vi "SteuerungWaermepumpe - Kopie_11.01.17.vi"() -> ()   [LabVIEW 2015]
uses:
  <vilib>/DAQmx/read.llb/DAQmx Read (Analog 1D Wfm NChan NSamp).vi
  <vilib>/DAQmx/write.llb/DAQmx Write (Analog 1D Wfm NChan 1Samp).vi
  <vilib>/MakerHub/LINX/Public/Peripherals/Digital/Digital Write N Chans.vi
  <vilib>/MakerHub/LINX/Private/Local IO/LinxDigitalWrite.vi
  <vilib>/MakerHub/LINX/Public/Utilities/Check Channel.vi
  <vilib>/MakerHub/LINX/Private/Utilties/Generate Error.vi
  <vilib>/DAQmx/miscellaneous.llb/DAQmx Fill In Error Info.vi
  <vilib>/Utility/file.llb/Read Delimited Spreadsheet (DBL).vi
  <vilib>/MakerHub/LINX/LMH-LINX.lvlib
panel:
  out "Array 2":waveform(dbl)[](array[waveform])
  in  "Messplatten speichern":bool caption="Enable"
  in  "Wartezeit 2":u32=500
  in  "Wartezeit 1":u32=9000
  out "Abscheider":cluster{dbl, dbl, dbl}(slide) scale=0.0..1.3
  in  "Rampe":bool=TRUE
  in  "Rampe rpm/s":dbl=1.0 min=1.0 max=100.0 step=1.0
  out "Rampe IW":dbl
  in  "reinitialize HD":bool
  in  "reinitialize Pumpe":bool
  out "ist an!":string
  in  "zusätzlicher Druck":dbl
  in  "PI05 SW":dbl format="%.2f"
  out "p_liq_mittel":dbl
  out "p_liq":dbl
  out "Schleifendauer":dbl format="%.5f"
  out "Mittelwert 2":dbl
  in  "Mittelwert HD":bool
  in  "Mittelwert Pumpe":bool
  out "Mittelwert":dbl
  in  "Xi / p_liq berechnung an":bool
  out "xi_r":dbl
  in  "Regler Senke":bool
  in  "reinitialize Senke":bool
  in  "TI35 SW":dbl=43.0 format="%.2f"
  in  "Drehzahl Bestätigung":bool
  in  "Drehzahl SW":dbl=1000.0 min=500.0 max=3000.0 step=1.0 format="%#_4g"
  out "Check":dbl format="%#_13g"
  in  "Regler Hochdruck":bool
  in  "PID Regelung Pumpe":bool
  in  "SW TI39":dbl
  out "Array":bool[](array[boolean])
  in  "LEDs 2":bool[](array[boolean])
  in  "Regelung HK":bool
  in  "RV 30 zu":bool
  in  "RV 30 auf":bool
  out "FI_Oel":dbl
  in  "RV 33":dbl(slide) scale=-1.0..1.0
  in  "tag":string
  out "Pumpenwerte":dbl[](array[numeric]) format="%.2f"
  out "Speichert!":bool
  out "Historie":string
  in  "Kommentar":string
  out "refnum out":refnum<file>
  in  "Identität!":string(combo)
  in  "Zeit X in Minuten":dbl(slide)=5.0 min=0.0 max=15.0 scale=5.0..15.0
  out "TI 21a Warnungen":dbl
  out "Leistung":dynamicdata(graph)
  out "TI 37":dbl
  in  "Programm stoppen!":bool
  out "%":sgl(slide) scale=0.0..100.0
  out "kalt":bool
  out "warm":bool
  out "?":T1(array[cluster]) {"?" format="%#.4g"; "Konzentration_reich" format="%#.4g"}
  in  "Mit EES vergleichen":bool
  in  "FI13 SW in l/min":dbl=3.0 min=3.0 max=12.0 step=0.10000000149011612
  out "COP_Oel":dbl
  out "Q-Oel kW":dbl format="%_4g"
  in  "Dateiname!":string
  in  "Comment":bool
  in  "Speichern":bool caption="Aktivieren"
  out "ZU     Ventilstellung 33     AUF":dbl(slide) scale=0.0..100.0 scale format="%.2f"
  in  "Regelventil 34":dbl(slide) min=0.0 max=100.0 step=0.009999999776482582 scale=0.0..100.0
  in  "Matlab":bool
  in  "?":T2(tab)
  out "?":dynamicdata(graph)
  out "?":waveform(dbl)(graph)
  out "?":dynamicdata(graph)
  out "PI 12":dbl format="%.2f"
  out "PI 11":dbl format="%.2f"
  out "Dichte":dbl format="%.5g"
  in  "Reset":bool
  out "Betriebszeit":cluster{"second":i32, "minute":i32, "hour":i32}
  out "Temperatur Ölprüfstand":dbl
  out "FI 13 kg/min":dbl
  in  "Messung\nFrequenzwandler":bool
  out "Magnetventil":bool
  out "Fl.Pumpe an":bool
  out "Temperatur Öl":bool
  out "COP":dbl format="%#_13g"
  out "Verdichteraktivität":cluster{"second":i32, "minute":i32, "hour":i32}
  out "Q-Entgaser kW":dbl format="%_4g"
  out "Warnungen":bool[](array[boolean])
  out "Status Komponenten":bool[](array[boolean])
  in  "Pumpen-Auto-Abschalt":bool=TRUE
  out "Q-Resorber kW":dbl format="%_4g"
  out "Stellung Expansionsventil":waveform(dbl)(graph)
  out "FI 35 l/min":dbl format="%#_13g"
  out "FI 38 l/min":dbl format="%#_13g"
  out "FI Oel l/min":dbl format="%#.3g"
  out "LI in l":dbl format="%#_4g"
  out "TI 39":dbl format="%#_3g"
  out "TI 38":dbl format="%#_3g"
  out "TI 36":dbl format="%#_3g"
  out "TI 35":dbl format="%#_3g"
  out "TI 33":dbl format="%#_3g"
  out "TI 32":dbl format="%#_3g"
  out "TI 34":dbl format="%#_3g"
  out "TI 21a":dbl format="%#_3g"
  out "TI 21":dbl format="%#_3g"
  out "TI 20":dbl format="%#_3g"
  out "TI 14a":dbl format="%#_3g"
  out "TI 14":dbl format="%#_3g"
  out "TI 13":dbl format="%#_3g"
  out "TI 12":dbl format="%#_3g"
  out "TI 11":dbl format="%#_3g"
  out "TI 10":dbl format="%#_3g"
  out "TI 09":dbl format="%#_3g"
  out "TI 08":dbl format="%#_3g"
  out "TI 07":dbl format="%#_3g"
  out "TI 06a":dbl format="%#_3g"
  out "TI 06":dbl format="%#_3g"
  out "TI 05":dbl format="%#_3g"
  out "TI 04":dbl format="%#_3g"
  out "TI 22":dbl format="%#_3g"
  out "TI 02":dbl format="%#_3g"
  out "TI 01":dbl format="%#_3g"
  out "Konzentration":dbl format="%#_5g"
  in  "Pumpensteuerung":dbl min=0.0 max=10.0 step=0.009999999776482582 format="%.2g"
  out "PI 08":dbl format="%.2f"
  out "PI 05":dbl format="%#.2f"
  out "PI 02":dbl format="%.2f"
  out "PI 04":dbl format="%.2f"
  out "PDI 8-9":dbl format="%.2f"
  out "PI 14":dbl format="%.2f"
  out "PI 01":dbl format="%.2f"
  out "ZU    Ventilstellung Exp.V     AUF":dbl(slide) scale=0.0..100.0 scale format="%#.1f"
  in  "Exp.V":dbl(slide)=3.0 min=0.0 max=100.0 step=1.0 scale=0.0..100.0 scale format="%#.0f"
  out "ZU    Ventilstellung 14      AUF":dbl(slide) caption="Auf    Ventilstellung 14      Zu" scale=0.0..100.0 scale format="%#.2f"
  in  "Regelventil 36":dbl(slide) min=0.0 max=100.0 step=0.009999999776482582 scale=0.0..100.0 scale format="%#.0f"
  out "ZU  Ventilstellung 35  AUF":dbl(slide) scale=0.0..100.0 scale format="%.2f"
  in  "Regelventil 35":dbl(slide)=100.0 min=0.0 max=100.0 step=0.009999999776482582 scale=0.0..100.0 scale format="%#.3g"
  out "ZU     Ventilstellung 39     AUF":dbl(slide) scale=0.0..100.0 scale format="%.2f"
  in  "Regelventil 39":dbl(slide)=100.0 min=0.0 max=100.0 step=0.009999999776482582 scale=0.0..100.0
  out "FI 13 l/min":dbl format="%.2f"
  out "FI 07 l/min":dbl format="%.2f"
  out "LI in m":dbl format="%.2f"
  out "PDI 5-6":dbl format="%.4f"
  out "PI 07":dbl format="%.2f"
  out "Druckverhältnis":dbl
  out "Drehzahl":dbl
  out "Drehmoment":dbl
  out "Frequenz":dbl
  out "Leistung":dbl
  out "Durchfluss":waveform(dbl)[](graph)
  in  "Tab Control Temperaturen":T3(tab)
  out "Temperatur Reich":waveform(dbl)[](graph)
  out "Temperatur Arm":waveform(dbl)[](graph)
  out "Temperatur Öl":waveform(dbl)[](graph)
  out "Temperatur Senke/Quelle":waveform(dbl)[](graph)
  out "Druck":waveform(dbl)[](graph)
  out "Druckzustand":bool caption="Zu viel Druck !!!"
  # "Öltemperatur"
  # "Resorber"
  # "Entgaser"
  # "Druckverhältnis"
  # "ExpV"
  # "Verdichter an"
  # "iWÜ"
  # "Magnetventil"
  # "RV 39"
  # "Leer"
  # "RV 33"
  # "RV 35"
  # "RV 34"
  # "Pumpe an"
  # "Ölabscheider"
  # "2"
  # "1"
  # "RV 30"
  # "Verdichter"
  # "Pumpe"
  # "Leistung"
  # "kW"
  # "Speed"
  # "rpm"
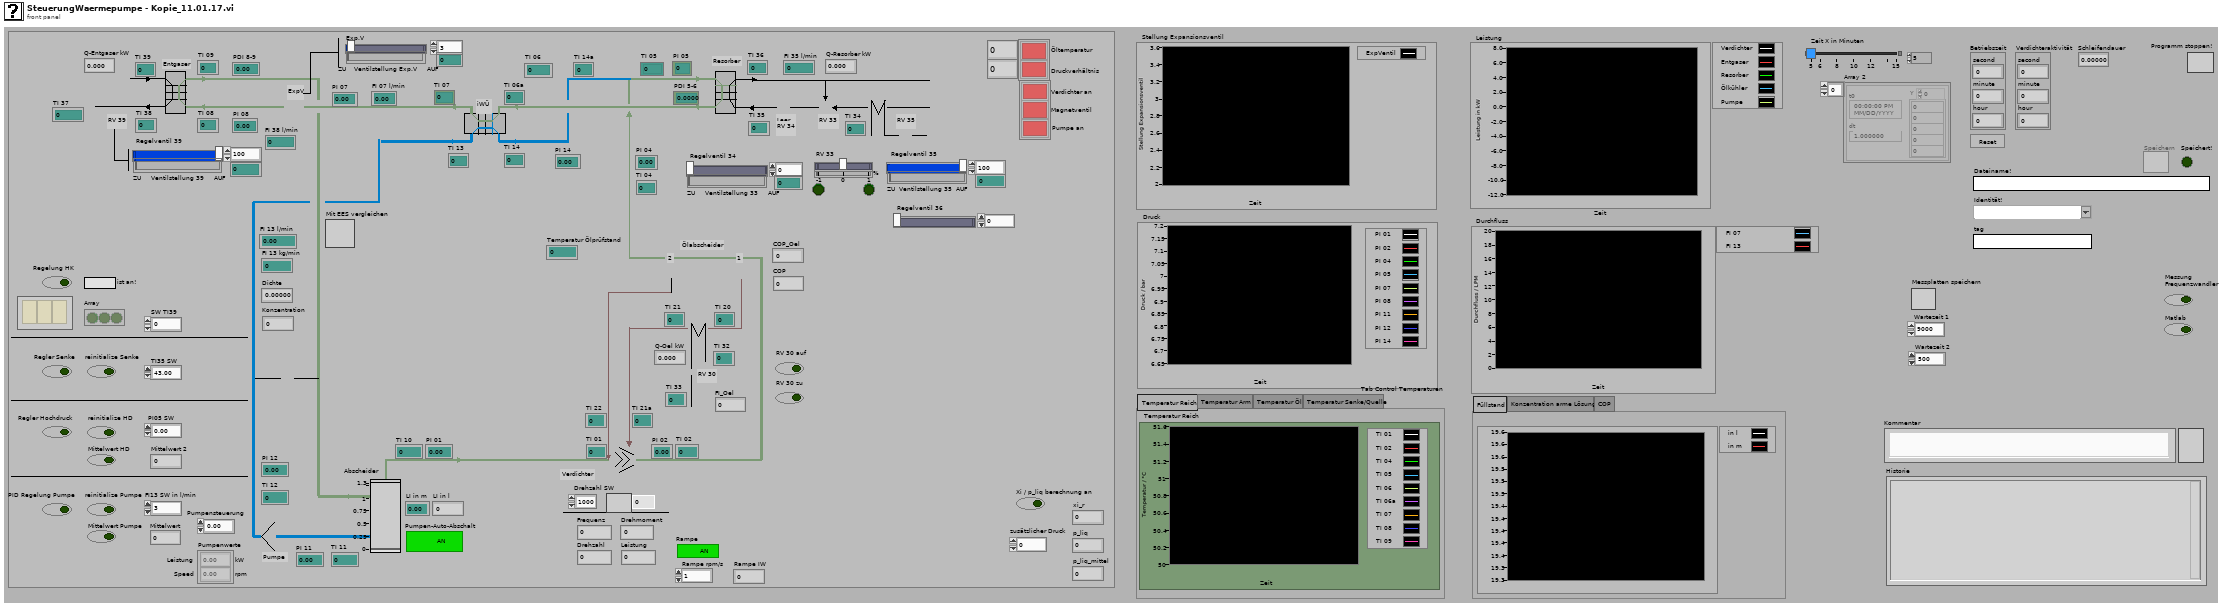
[diagram p1: front panel]
types:
  T1 = cluster{dbl, "Konzentration_reich":dbl, "String":string, bool}[]
  T2 = enum32{"Füllstand", "Konzentration arme Lösung", "COP"}
  T3 = enum32{"Temperatur Reich", "Temperatur Arm", "Temperatur Öl", "Temperatur Senke/Quelle"}
  T4 = enum8{"Enabled", "Disabled", "Disabled and Grayed Out"}
  T5 = typedef "LMH-LINX.lvlib/LINX Ref.ctl" = cluster{"IO":T6, "Interface":T7, "LINX Device Config":T8}
  T6 = typedef "LMH-LINX.lvlib/Platform.ctl" = enum16{"Remote", "Local"}
  T7 = typedef "LMH-LINX.lvlib/Interface.ctl" = enum16{"Serial", "TCP"}
  T8 = typedef "LMH-LINX.lvlib/Device.lvlib/LINX Device Config.ctl" = cluster{"Interface":T7, "COM Port":refnum<visa-resource-name>, "TCP Configuration":T9, "Device Family":u8, "Device ID":u8, "Device Name":string, "TCP Ref":refnum<k5>, "Channels":T10}
  T9 = typedef "LMH-LINX.lvlib/Device.lvlib/TCP Config.ctl" = cluster{"IP Address":string, "Port":u16}
  T10 = typedef "LMH-LINX.lvlib/Channels.ctl" = cluster{"DI":u8[], "DO":u8[], "AI":u8[], "AO":u8[], "PWM":u8[], "QE":u8[], "UART":u8[], "I2C 2":u8[], "SPI":u8[], "CAN":u8[], "Servo":u8[], "AI Ref (V)":dbl, "AI Resolution (Bits)":u8, "AO Ref (V)":dbl, "AO Resolution (Bits)":u8}
  T11 = enum16{"open", "replace", "create", "open or create", "replace or create", "replace or create with confirmation"}
  T12 = cluster{"Array[0]":dbl, "Array[1]":dbl, "Array[2]":dbl}
  T13 = cluster{"Array[0]":sgl, "Array[1]":sgl, "Array[2]":sgl}
  T14 = cluster{"Numeric":dbl, "Konzentration_reich":dbl, "String":string, bool}[]
  T15 = typedef "LVDateTimeRec.ctl" = cluster{"fractional second":dbl, "second":i32, "minute":i32, "hour":i32, "day of month":i32, "month":i32, "year":i32, "day of week":i32, "day of year":i32, "DST":i32}
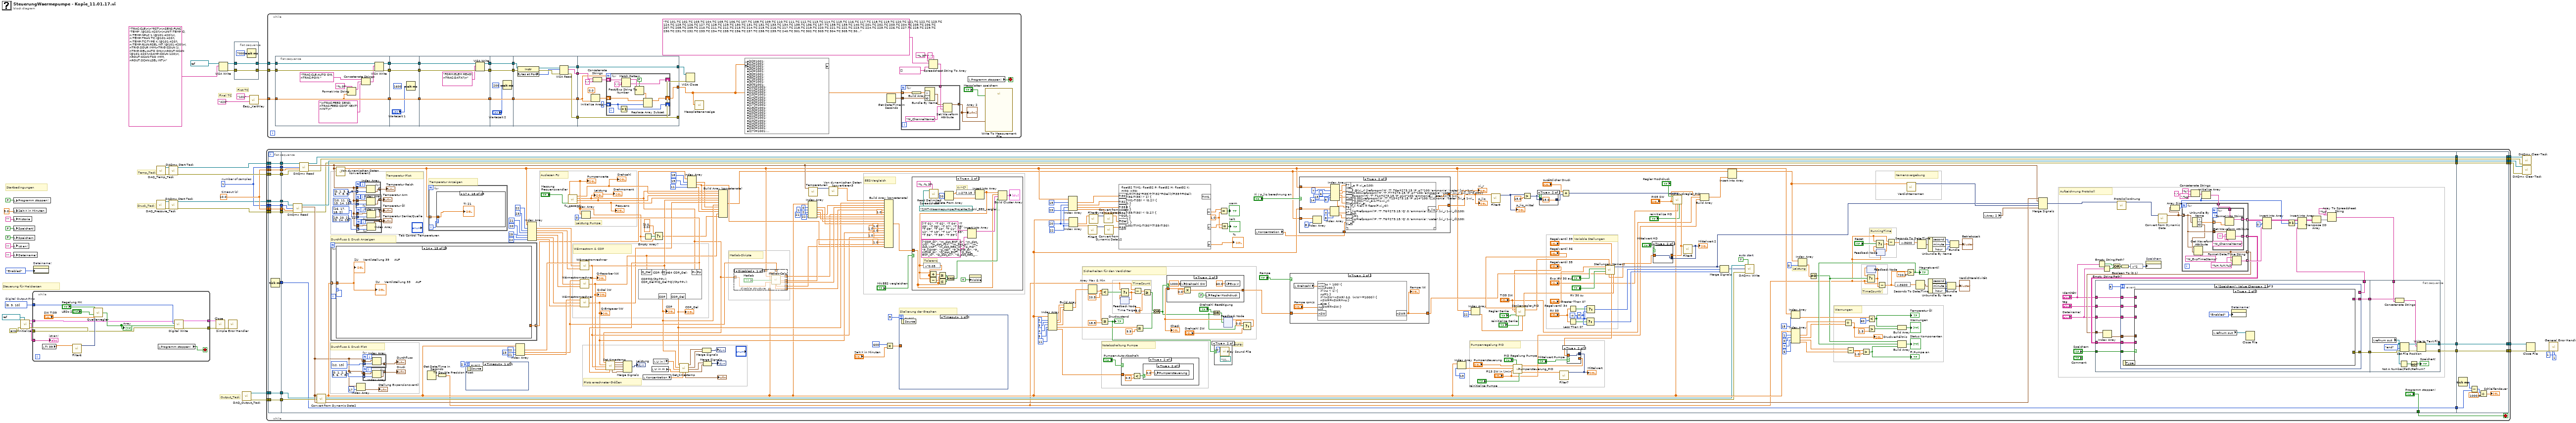
[diagram p0: block diagram]
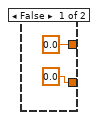
[diagram p8: hidden frame]
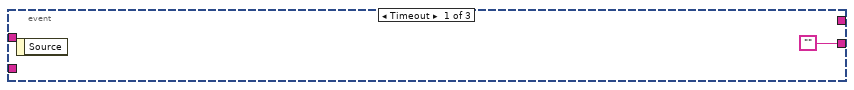
[diagram p10: hidden frame]
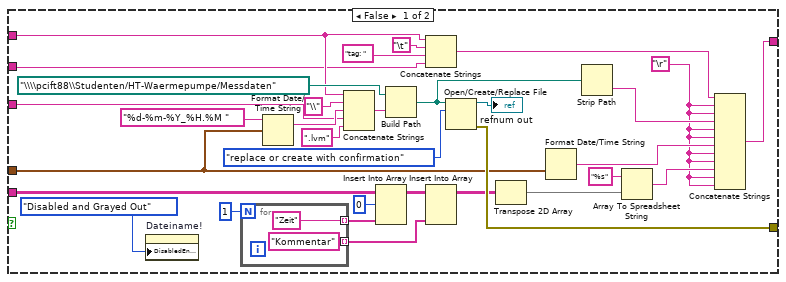
[diagram p11: hidden frame]
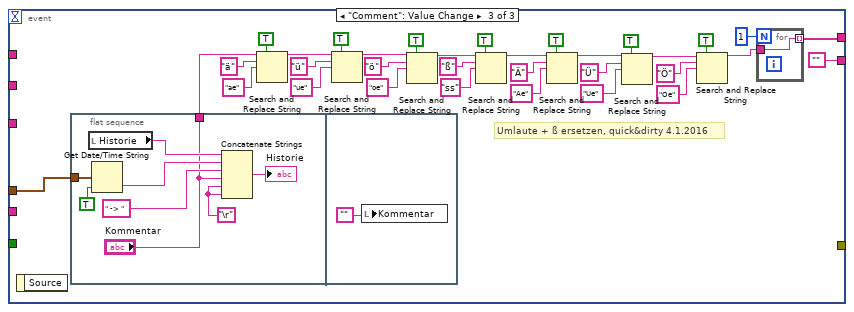
[diagram p12: hidden frame]
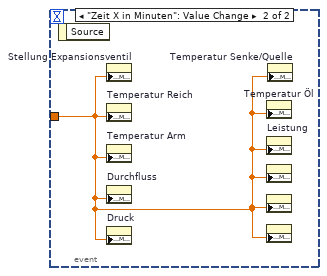
[diagram p13: hidden frame]
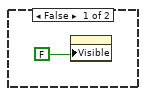
[diagram p14: hidden frame]
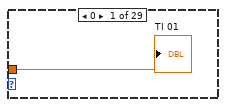
[diagram p17: hidden frame]
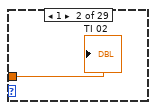
[diagram p18: hidden frame]
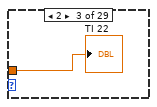
[diagram p19: hidden frame]
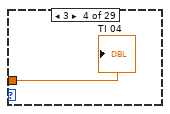
[diagram p20: hidden frame]
diagram:
  w19 = 10.0  # timeout (s)
  w18 = 1  # number of samples
  w31 = i32[] [8, 9, 10]  # Digital Output PIns
  # "Final TC"
  # "First TC"
  # "Output_Task"
  # "Druck_Task"
  # "Temp_Task"
  # "Steuerung für Heizkerzen"
  # "Startbedingungen"
  n1 = local write "Programm stoppen!"(FALSE ("Programm stoppen!")) -> ()
  n2 = local write "Zeit X in Minuten"(5.0 ("Zeit X in Minuten")) -> ()
  n3 = local write "Historie"("") -> ()
  n4 = local write "Speichert!"(FALSE ("Speichert!")) -> ()
  n5 = local write "Speichern"(FALSE ("Speichern")) -> ()
  n6 = local write "ist an!"("") -> ()
  n7 = local write "Dateiname!"("") -> ()
  n8 = call <vilib>:"Initialize.vi"("Serial Port"=refnum<visa-resource-name> "COM4", "Error In"=errorcluster {"status"=FALSE, "code"=0, "source"=""}) -> ("Error Out"=w32:errorcluster, "Device Name"=w29:string, "LINX Resource"=w35:T5)  [unwired: 7 in]
  n9 = while {
    tunnel: w35 -> [w50]
    tunnel: [w60] -> w34
    tunnel: [w59] -> w33
    tunnel: w32 -> [w49]
    tunnel: w31 -> [w58]
    tunnel: w29 -> [w48]
    stop <- w57 stop-if-true
    n10 = local read "TI 39"() -> (w51:dbl)
    n11 = call "Filter6"("Signal"=w51) -> ("Filtered Signal"=w52:dynamicdata)  [unwired: 9 in, 1 out]
    n12 = call "Quellenregler.vi"("Regelung Quelle"="Regelung HK", "TI 38 IW °C"=w52, "LEDs"="LEDs 2", "TI 38 SW °C"="SW TI39") -> ("Kerzen von Regler"=w54:bool[])  [unwired: 3 in, 1 out]
    "Array" <- w54
    n13 = local read "Programm stoppen!"() -> (w57:bool)
    n14 = call-poly <vilib>:"Digital Write.vi"("Error In"=w49, "Values"=w54, "DO Channels"=w58, "LINX Resource"=w50) -> ("Error Out"=w59:errorcluster, "LINX Resource"=w60:T5)  [unwired: 6 in]
    "ist an!" <- w48
  }
  n15 = property on="Dateiname!" class="Str"("DisabledEnum"=T4."Enabled" ("Disabled")) -> ()  [unwired: 2 in, 2 out]
  n16 = call "DAQ_Pressure_Task.vi"() -> ("error out"=w23:errorcluster, "task out"=w24:refnum<k21>)  [unwired: 10 in]
  n17 = call "DAQ_Temp_Task.vi"() -> ("error out"=w25:errorcluster, "task out"=w26:refnum<k21>)  [unwired: 10 in]
  n18 = call <vilib>:"DAQmx Start Task.vi"("task/channels in"=w24, "error in"=w23) -> ("task out"=w17:refnum<k21>, "error out"=w20:errorcluster)  [unwired: 12 in]
  n19 = call <vilib>:"DAQmx Start Task.vi"("task/channels in"=w26, "error in"=w25) -> ("task out"=w21:refnum<k21>, "error out"=w22:errorcluster)  [unwired: 12 in]
  n20 = call <vilib>:"Close.vi"("Error In"=w33, "LINX Resource"=w34) -> ("Error Out"=w36:errorcluster)  [unwired: 9 in]
  n21 = VISA Write(VISA resource name=refnum<visa-resource-name> "COM3", write buffer="TRAC:CLE\n\n*RST\n\nSENS:FUNC 'TEMP',(@101:420)\n\nUNIT:TEMP C\n:TEMP:NPLC 1,(@101:420)\n\n:TEMP:TRAN TC,(@101:420)\n:TEMP:TC:TYPE K,(@101:420)\n:TEMP:RJUN:RSEL INT,(@101:420)\n\nTRIG:SOUR IMM\nTRIG:COUN 1\nTRIG:DEL:AUTO ON\n\nROUT:SCAN  (@101:420)\nSAMP:COUN 120\n\nROUT:SCAN:TSO IMM\nROUT:SCAN:LSEL INT\n") -> (VISA resource name out=w5:refnum<visa-resource-name>, error out=w6:errorcluster)  [unwired: 1 in, 1 out]
  n22 = call <vilib>:"Simple Error Handler.vi"("error in (no error)"=w36) -> ()  [unwired: 4 in, 5 out]
  n23 = flat-sequence {
    tunnel: w6 -> [w63]
    tunnel: [w63] -> w3
    tunnel: w5 -> [w61]
    tunnel: [w61] -> w4
    frame #0 {
      n24 = Wait (ms)(milliseconds to wait=u32 7000 ("Zu wartende ms")) -> ()  [unwired: 1 out]
    }
  }
  n25 = call "DAQ_Output_Task.vi"() -> ("error out"=w11:errorcluster, "task out"=w12:refnum<k21>)  [unwired: 10 in]
  n26 = call "Easy_Keithley.vi"("Final Thermocouple ID# (String)"="420", "First Thermocouple ID# (String)"="101") -> ("Number of Thermocouples"=w7:dbl)  [unwired: 8 in, 1 out]
  n27 = while {
    tunnel: [w98] -> w41
    tunnel: [w97] -> w40
    tunnel: w22 -> [w91]
    tunnel: w19 -> [w89]
    tunnel: w21 -> [w86]
    tunnel: w18 -> [w84]
    tunnel: w20 -> [w82]
    tunnel: w19 -> [w81]
    tunnel: w18 -> [w79]
    tunnel: w17 -> [w77]
    tunnel: [w73] -> w16
    tunnel: [w72] -> w15
    tunnel: [w70] -> w14
    tunnel: [w68] -> w13
    tunnel: w12 -> [w67]
    tunnel: w11 -> [w64]
    stop <- w96 stop-if-true
    n28 = flat-sequence {
      tunnel: [w109] -> w92
      tunnel: w91 -> [w108]
      tunnel: [w108] -> w90
      tunnel: w89 -> [w107]
      tunnel: [w107] -> w88
      tunnel: w86 -> [w106]
      tunnel: [w106] -> w87
      tunnel: [w105] -> w85
      tunnel: w84 -> [w105]
      tunnel: [w104] -> w83
      tunnel: w82 -> [w104]
      tunnel: w81 -> [w103]
      tunnel: [w103] -> w80
      tunnel: w79 -> [w102]
      tunnel: [w102] -> w78
      tunnel: w77 -> [w101]
      tunnel: [w101] -> w76
      tunnel: w67 -> [w100]
      tunnel: [w100] -> w66
      tunnel: [w99] -> w65
      tunnel: w64 -> [w99]
      tunnel: ["Programm stoppen!"] -> w96
      tunnel: [w327] -> w95
      tunnel: [w326] -> w94
      tunnel: [w131] -> w93
      tunnel: w92 -> [w131]
      tunnel: w90 -> [w168]
      tunnel: w88 -> [w167]
      tunnel: w87 -> [w166]
      tunnel: w85 -> [w165]
      tunnel: w83 -> [w164]
      tunnel: w80 -> [w163]
      tunnel: w78 -> [w162]
      tunnel: w76 -> [w161]
      tunnel: [w160] -> w75
      tunnel: [w159] -> w74
      tunnel: [w158] -> w71
      tunnel: [w157] -> w69
      tunnel: w66 -> [w155]
      tunnel: w65 -> [w154]
      tunnel: [w738] -> w97
      tunnel: [w739] -> w98
      tunnel: w95 -> [w739]
      tunnel: w94 -> [w738]
      tunnel: w93 -> [w736]
      tunnel: w75 -> [w731]
      tunnel: w74 -> [w732]
      tunnel: [w732] -> w73
      tunnel: [w731] -> w72
      tunnel: w71 -> [w730]
      tunnel: [w730] -> w70
      tunnel: w69 -> [w729]
      tunnel: [w729] -> w68
      frame #0 {
        n29 = Tick Count (ms)() -> (millisecond timer value=w109:u32)
      }
      frame #1 {
        w133 = 8.0  # Time Target
        w156 = TRUE  # auto start
        w347 = sgl 1.0
        w360 = 22
        w365 = 20
        w391 = -4
        w392 = 0
        # "RunningTime"
        # "TimeCountV"
        # "TimeCount"
        # "ENTE!"
        # "Sicherheiten für den Verdichter"
        # "Pumpenregelung PID"
        # "Skalierung der Graphen"
        # "Leistung Pumpe"
        # "Leistung"
        # "Durchfluss & Druck Anzeigen"
        # "Temperatur Anzeigen"
        # "Plots errechneter Größen"
        # "EES-Vergleich"
        # "Matlab-Skripte"
        # "Warnungen"
        # "Namensvergebung"
        # "Wärmestrom & COP"
        # "Notabschaltung Pumpe"
        # "Auslesen FU"
        # "Durchfluss & Druck Plot"
        # "Temperatur Plot"
        # "Aufzeichnung Protokoll"
        # "Variable Stellungen"
        n30 = call-poly <vilib>:"DAQmx Read.vi"("task/channels in"=w161, "number of samples per channel"=w162, "timeout"=w163, "error in"=w164) -> ("task out"=w160:refnum<k21>, "data"=w170:waveform(dbl)[], "error out"=w157:errorcluster)  [unwired: 9 in]
        n31 = call-poly <vilib>:"DAQmx Read.vi"("task/channels in"=w166, "number of samples per channel"=w165, "timeout"=w167, "error in"=w168) -> ("task out"=w159:refnum<k21>, "data"=w169:waveform(dbl)[], "error out"=w158:errorcluster)  [unwired: 9 in]
        n32 = call "Convert from Dynamic Data2"("Dynamic Data Type"=w170) -> ("Array"=w175:dbl[])  [unwired: 3 in]
        n33 = for {
          tunnel: w175 -> [w677] mode=indexing
          tunnel: [w676] -> w180 mode=indexing
          i -> [w678]
          n34 = case shown="14" w678 {
            tunnel: w677 -> [w679 w680 w681 w682 w683 w684 w685 w686 w687 w688 w689 w698 w710 w713 w714 w715 w716 w717 w720 w724 w725 w726 w727 w728 _]
            tunnel: [_ _ _ _ _ _ _ _ _ _ _ w690 _ _ _ _ _ _ w718 w722 _ _ _ _ _] -> w676
            frame 0 {
              "PI 01" <- w679
            }
            frame 1 {
              "PI 02" <- w680
            }
            frame 2 {
              "PI 04" <- w681
            }
            frame 3 {
              "PI 05" <- w682
            }
            frame 4 {
              "PI 07" <- w683
            }
            frame 5 {
              "PI 08" <- w684
            }
            frame 6 {
              "PI 11" <- w685
            }
            frame 7 {
              "PI 12" <- w686
            }
            frame 8 {
              "PI 14" <- w687
            }
            frame 9 {
              "PDI 5-6" <- w688
            }
            frame 10 {
              "PDI 8-9" <- w689
            }
            frame 11 {
              n35 = call "Filter3"("Signal"=w698) -> ("Filtered Signal"=w696:dynamicdata)  [unwired: 9 in, 1 out]
              n36 = Greater?(x=w698, y=0.3) -> (0:w693:bool)
              n37 = case shown="False" w693 {
                tunnel: w698 -> [_ w709]
                tunnel: [0.0 w709] -> w701
                frame False {
                }
                frame True {
                }
              }
              n38 = call "Convert from Dynamic Data6"("Dynamic Data Type"=w696) -> ("Scalar"=w695:dbl)  [unwired: 3 in]
              n39 = Multiply(x=w695, y=10.0) -> (x*y=w697:dbl)
              n40 = Greater?(x=w698, y=0.4) -> (0:w694:bool)
              n41 = formula code="float64 y; float64 Vu; /*Vu: Volumen schmaler Zylinder+Fuellstandsmesser*/\nVu=10;  /* 10 Liter */\n\nif (x<=10.25) \ny=(x-1)*pi*(0.536**2+0.32**2);\nelse\ny=Vu+(x-10.25)*pi*(1.584**2+0.32**2);"("x"=w697) -> ("y"=w690:dbl)
              "LI in l" <- w690
              n42 = case shown="False" w694 {
                tunnel: w698 -> [_ w707]
                tunnel: [0.0 w707] -> w700
                frame False {
                }
                frame True {
                }
              }
              n43 = Merge Signals(w698, w701, w700) -> (w702:dynamicdata)
              n44 = call "Convert from Dynamic Data3"("Dynamic Data Type"=w702) -> ("Array"=w705:dbl[])  [unwired: 3 in]
              n45 = Array To Cluster(array=w705) -> (cluster=w692:T12)
              n46 = To Single Precision Float(number=w692) -> (single precision float=→"Abscheider":T13)
              "LI in m" <- w698
            }
            frame 12 {
              "FI 07 l/min" <- w710
            }
            frame 13 {
              n47 = local read "Dichte"() -> (w712:dbl)
              n48 = Multiply(x=w713, y=w712) -> (x*y=→"FI 13 kg/min":dbl)
              "FI 13 l/min" <- w713
            }
            frame 14 {
              "ZU     Ventilstellung 39     AUF" <- w714
              "ZU     Ventilstellung 33     AUF" <- w714
            }
            frame 15 {
              "ZU  Ventilstellung 35  AUF" <- w715
            }
            frame 16 {
              # "RV14 ist entfernt"
              "ZU    Ventilstellung 14      AUF" <- w716
            }
            frame 17 {
              "ZU    Ventilstellung Exp.V     AUF" <- w717
            }
            frame 18 {
              n49 = call "Filter"("Signal"=w720) -> ("Filtered Signal"=w719:dynamicdata)  [unwired: 9 in, 1 out]
              n50 = call "Convert from Dynamic Data4"("Dynamic Data Type"=w719) -> ("Scalar"=w721:dbl)  [unwired: 3 in]
              n51 = formula code="float64 D;\nD=9.375*StromDichte+0.7125;\nD=floor(D*100000)/100000;"("StromDichte"=w721) -> ("D"=w718:dbl)
              "Dichte" <- w718
            }
            frame 19 {
              n52 = call "Filter2"("Signal"=w724) -> ("Filtered Signal"=w723:dynamicdata)  [unwired: 9 in, 1 out]
              n53 = To Double Precision Float(number=w723) -> (double precision float=w722:dbl)
              "Konzentration" <- w722
            }
            frame 20 {
              "FI Oel l/min" <- w725
            }
            frame 21 {
              "FI 38 l/min" <- w726
            }
            frame 22 {
              "FI 35 l/min" <- w727
            }
            frame 23 {
              "FI_Oel" <- w728
            }
            frame 24, Default {
            }
          }
        }
        n54 = call "Von dynamischen Daten konvertieren2"("Dynamic Data Type"=w169) -> ("Array"=w116:dbl[])  [unwired: 3 in]
        n55 = for {
          tunnel: i32[] [0, 1, 3, 4, 5, 6, 7, 8, 9] -> [w491] mode=indexing
          tunnel: w169 -> [w490]
          tunnel: [w489] -> w263 mode=indexing
          n56 = Index Array(array=w490, index=w491) -> (element=w489:waveform(dbl))
        }
        "Temperatur Reich" <- w263
        n57 = for {
          tunnel: i32[] [10, 11, 12, 13, 14, 15] -> [w488] mode=indexing
          tunnel: w169 -> [w487]
          tunnel: [w486] -> w264 mode=indexing
          n58 = Index Array(array=w487, index=w488) -> (element=w486:waveform(dbl))
        }
        "Temperatur Arm" <- w264
        n59 = for {
          tunnel: i32[] [16, 17, 18, 2] -> [w485] mode=indexing
          tunnel: w169 -> [w484]
          tunnel: [w483] -> w265 mode=indexing
          n60 = Index Array(array=w484, index=w485) -> (element=w483:waveform(dbl))
        }
        "Temperatur Öl" <- w265
        n61 = Index Array(array=w170, index=17) -> (element=→"Stellung Expansionsventil":waveform(dbl))
        n62 = for {
          tunnel: i32[] [19, 20, 21, 22, 23, 24, 25] -> [w482] mode=indexing
          tunnel: w169 -> [w481]
          tunnel: [w480] -> w266 mode=indexing
          n63 = Index Array(array=w481, index=w482) -> (element=w480:waveform(dbl))
        }
        "Temperatur Senke/Quelle" <- w266
        n64 = for {
          tunnel: [w476] -> w261 mode=indexing
          tunnel: w170 -> [w475]
          tunnel: i32[] [0, 1, 2, 3, 4, 5, 6, 7, 8] -> [w474] mode=indexing
          n65 = Index Array(array=w475, index=w474) -> (element=w476:waveform(dbl))
        }
        "Druck" <- w261
        n66 = for {
          tunnel: [w479] -> w262 mode=indexing
          tunnel: w170 -> [w478]
          tunnel: i32[] [12, 13] -> [w477] mode=indexing
          n67 = Index Array(array=w478, index=w477) -> (element=w479:waveform(dbl))
        }
        "Durchfluss" <- w262
        n68 = Get Date/Time In Seconds() -> (seconds since 1Jan1904=w130:timestamp)
        n69 = for {
          tunnel: w116 -> [w646] mode=indexing
          i -> [w647]
          n70 = case shown="17" w647 {
            tunnel: w646 -> [w648 w649 w650 w651 w652 w653 w654 w655 w656 w657 w658 w659 w660 w661 w662 w663 w664 w665 w666 w667 w668 w669 w670 w671 w672 w673 w674 w675 _]
            frame 0 {
              "TI 01" <- w648
            }
            frame 1 {
              "TI 02" <- w649
            }
            frame 2 {
              "TI 22" <- w650
            }
            frame 3 {
              "TI 04" <- w651
            }
            frame 4 {
              "TI 05" <- w652
            }
            frame 5 {
              "TI 06" <- w653
            }
            frame 6 {
              "TI 06a" <- w654
            }
            frame 7 {
              "TI 07" <- w655
            }
            frame 8 {
              "TI 08" <- w656
            }
            frame 9 {
              "TI 09" <- w657
            }
            frame 10 {
              "TI 10" <- w658
            }
            frame 11 {
              "TI 11" <- w659
            }
            frame 12 {
              "TI 12" <- w660
            }
            frame 13 {
              "TI 13" <- w661
            }
            frame 14 {
              "TI 14" <- w662
            }
            frame 15 {
              "TI 14a" <- w663
            }
            frame 16 {
              "TI 20" <- w664
            }
            frame 17 {
              "TI 21" <- w665
            }
            frame 18 {
              "TI 21a" <- w666
              "TI 21a Warnungen" <- w666
            }
            frame 19 {
              # "Check T_Heater"
              "TI 34" <- w667
            }
            frame 20 {
              "TI 32" <- w668
            }
            frame 21 {
              "TI 33" <- w669
            }
            frame 22 {
              "TI 35" <- w670
            }
            frame 23 {
              "TI 36" <- w671
            }
            frame 24 {
              "TI 38" <- w672
            }
            frame 25 {
              "TI 39" <- w673
            }
            frame 26 {
              "Temperatur Ölprüfstand" <- w674
            }
            frame 27 {
              "TI 37" <- w675
            }
            frame 28, Default {
            }
          }
        }
        n71 = To Double Precision Float(number=w130) -> (double precision float=w118:dbl)
        n72 = event shown="[0] Timeout" {
          selector: _ -> [_]
          dyn-events: _ -> [_]
          timeout: 2 -> [_]
          event Timeout {
            n73 = event-data() -> ()  [unwired: 1 in, 1 out]
          }
        }
        n74 = Index Array(array=w175, index #1=22 ("index"), index #2=23 ("index"), index #3=21 ("index")) -> (element #1=w296:dbl, element #2=w272:dbl, element #3=w295:dbl)
        n75 = Index Array(array=w116, index #1=22 ("index"), index #2=23 ("index"), index #3=21 ("index"), index #4=20 ("index"), index #5=25 ("index"), index #6=24 ("index")) -> (element #1=w294:dbl, element #2=w293:dbl, element #3=w292:dbl, element #4=w291:dbl, element #5=w290:dbl, element #6=w289:dbl)
        n76 = call "fu_gesamt.vi"("Boolean"="Messung\nFrequenzwandler") -> ("Frequenz"=w284:dbl, "Drehmoment"=w285:dbl, "Leistung"=w141:dbl, "Drehzahl"=w286:dbl, "Scaled"=w143:dbl[])  [unwired: 6 in]
        "Leistung" <- w141
        "Frequenz" <- w284
        "Drehmoment" <- w285
        "Drehzahl" <- w286
        "Pumpenwerte" <- w143
        n77 = call "Wärmestromrechner.vi"("Taus"=w293, "Tein"=w294, "Massenstrom"=w296) -> ("Wärmestrom Q"=w194:dbl)  [unwired: 2 in]
        "Q-Resorber kW" <- w194
        n78 = call "Wärmestromrechner.vi"("Taus"=w291, "Tein"=w292, "Massenstrom"=w272) -> ("Wärmestrom Q"=w181:dbl)  [unwired: 2 in]
        "Q-Oel kW" <- w181
        n79 = call "Wärmestromrechner.vi"("Taus"=w289, "Tein"=w290, "Massenstrom"=w295) -> ("Wärmestrom Q"=w193:dbl)  [unwired: 2 in]
        "Q-Entgaser kW" <- w193
        n80 = Index Array(array=w143, index=0) -> (element=w195:dbl)
        n81 = call "Set_timestamp.vi"("Eingang 5"=w195, "Eingang 4"=w181, "Eingang 3"=w194, "Eingang 2"=w193, "Eingang"=w141) -> ("Ausgang 4"=w191:waveform(dbl), "Ausgang 3"=w190:waveform(dbl), "Ausgang 2"=w189:waveform(dbl), "Ausgang"=w188:waveform(dbl), "Ausgang 5"=w192:waveform(dbl))  [unwired: 2 in]
        n82 = Merge Signals(w188, w189, w190, w191, w192) -> (→"Leistung":dynamicdata)
        n83 = formula code="float64 COP; float64 COP_Oel;\n\nCOP=Q/(Pp+Pv);\nCOP_Oel=(Q_Oel+Q)/(Pp+Pv);"("Pv"=w141, "Q"=w194, "Pp"=w195, "Q_Oel"=w181) -> ("COP"=w203:dbl, "COP_Oel"=w202:dbl)
        "COP" <- w203
        "COP_Oel" <- w202
        n84 = local read "Konzentration"() -> (w207:dbl)
        n85 = Empty Array?(array=w143) -> (empty?=w145:bool)
        n86 = local read "LI in m"() -> (w205:dbl)
        n87 = local read "LI in l"() -> (w204:dbl)
        n88 = Select(t=dbl[] [0.0, 0.0], s=w145, f=w143) -> (s? t:f=w142:dbl[])
        n89 = call "Set_timestamp.vi"("Eingang 5"=w207, "Eingang 4"=w205, "Eingang 3"=w204, "Eingang 2"=w203, "Eingang"=w202) -> ("Ausgang 4"=w200:waveform(dbl), "Ausgang 3"=w199:waveform(dbl), "Ausgang 2"=w197:waveform(dbl), "Ausgang"=w196:waveform(dbl), "Ausgang 5"=→"?":waveform(dbl))  [unwired: 2 in]
        n90 = Index Array(array=w180, index #1=18 ("index"), index #2=19 ("index"), index #3=11 ("index")) -> (element #1=w182:dbl, element #2=w179:dbl, element #3=w183:dbl)
        n91 = Merge Signals(w196, w197) -> (→"?":dynamicdata)
        n92 = Merge Signals(w199, w200) -> (→"?":dynamicdata)
        n93 = Build Array (concatenate)(w141, w286, w285, w284, w194, w193, w203, w182, w179, w183, w181, w142) -> (w115:dbl[])
        n94 = disable-structure shown="Disabled" {
          disable-tunnel: [w436 _] -> w388
          disable-tunnel: [w435 _] -> w377
          disable-tunnel: [w434 _] -> w366
          disable-tunnel: [w433 _] -> w288
          disable-tunnel: [w432 _] -> w283
          disable-tunnel: w272 -> [w431 _]
          disable-tunnel: w141 -> [w430 _]
          disable-tunnel: w175 -> [w429 _]
          disable-tunnel: w116 -> [w428 _]
          frame Disabled {
            n95 = call "Matlab-Calc.vi"("Temp-Array"=w428, "Matlab?"="Matlab", "Leistung"=w430, "Druck-Array"=w429, "FI Öl"=w431) -> ("m_reich [g/s]"=w435:dbl, "Konzentration_reich"=w432:dbl, "m_arm [g/s]"=w436:dbl, "Dampfmassenstrom [g/s]"=w433:dbl, "Dampfmassenanteil"=w434:dbl)  [unwired: 3 in, 7 out]
          }
          frame Enabled {
          }
        }
        n96 = Index Array(array=w175, index #1=0 ("index"), index #2=1 ("index"), index #3=2 ("index"), index #4=21 ("index"), index #5=22 ("index")) -> (element #1=w371:dbl, element #2=w372:dbl, element #3=w373:dbl, element #4=w370:dbl, element #5=w368:dbl)
        n97 = call "Temperaturen"("Signals"=w169) -> ("Signal Out"=w378:dynamicdata)  [unwired: 9 in, 1 out]
        n98 = call "Von dynamischen Daten konvertieren3"("Dynamic Data Type"=w378) -> ("Array"=w379:dbl[])  [unwired: 3 in]
        n99 = Build Array (concatenate)(w379, w202, w370, w388, w377, 1.0 ("element"), w288, w368, w373, w372, w371, 1.0 ("element"), 1.0 ("element"), 1.0 ("element"), w193, 1.0 ("element"), w194, w366, 1.0 ("element"), w179, w283) -> (w380:dbl[])
        n100 = Multiply(x=600, y="Zeit X in Minuten") -> (x*y=w339:dbl)
        n101 = event shown="[0] Timeout" {
          selector: _ -> [_ _]
          dyn-events: _ -> [_ _]
          timeout: 5 -> [_ _]
          tunnel: w339 -> [_ w620]
          event Timeout {
            n102 = event-data() -> ()  [unwired: 1 in, 1 out]
          }
          event "Zeit X in Minuten": Value Change {
            n103 = event-data() -> ()  [unwired: 1 in, 1 out]
            n104 = property on="Stellung Expansionsventil" class="WFChart (strict)"("XScale.Maximum"=w620) -> ()  [unwired: 2 in, 2 out]
            n105 = property on="Temperatur Reich" class="WFChart (strict)"("XScale.Maximum"=w620) -> ()  [unwired: 2 in, 2 out]
            n106 = property on="Temperatur Arm" class="WFChart (strict)"("XScale.Maximum"=w620) -> ()  [unwired: 2 in, 2 out]
            n107 = property on="Durchfluss" class="WFChart (strict)"("XScale.Maximum"=w620) -> ()  [unwired: 2 in, 2 out]
            n108 = property on="Druck" class="WFChart (strict)"("XScale.Maximum"=w620) -> ()  [unwired: 2 in, 2 out]
            n109 = property on="Temperatur Öl" class="WFChart (strict)"("XScale.Maximum"=w620) -> ()  [unwired: 2 in, 2 out]
            n110 = property on="Leistung" class="WFChart (strict)"("XScale.Maximum"=w620) -> ()  [unwired: 2 in, 2 out]
            n111 = property class="WFChart (strict)"("XScale.Maximum"=w620) -> ()  [unwired: 2 in, 2 out]
            n112 = property class="WFChart (strict)"("XScale.Maximum"=w620) -> ()  [unwired: 2 in, 2 out]
            n113 = property class="WFChart (strict)"("XScale.Maximum"=w620) -> ()  [unwired: 2 in, 2 out]
            n114 = property on="Temperatur Senke/Quelle" class="WFChart (strict)"("XScale.Maximum"=w620) -> ()  [unwired: 2 in, 2 out]
          }
        }
        n115 = case shown="True" "Mit EES vergleichen" {
          tunnel: w380 -> [_ w622]
          frame False {
            n116 = property class="Arr (strict)"("Visible"=FALSE) -> ()  [unwired: 2 in, 2 out]
          }
          frame True {
            # "K->C°"
            # "Toleranz"
            n117 = call-poly <vilib>:"Read Delimited Spreadsheet.vi"("file path (dialog if empty)"=path "Z:/HT-Waermepumpe/Projekte/SubVi_EES_vergleich/test.txt", "format (%.3f)"="%,;%.3f") -> ("first row"=w629:dbl[])  [unwired: 8 in, 5 out]
            n118 = Delete From Array(array=w629, length=20) -> (deleted portion=w625:dbl[], array with subset deleted=w627:dbl[])  [unwired: 1 in]
            n119 = expression code="x-273.15"(w627) -> (w626:dbl[])
            n120 = Insert Into Array(array=string[] ["T 01", "T 02", "T 04", "T 05", "T 06", "T 07", "T 08", "T 09", "T 10", "T 11", "T 12", "T 13", "T 14", "T 35", "T 36", "T 38", "T 39"] ("Array"), new element=string[] ["COP_Öl", "m_dot_ENT_W", "m_dot_LIQ", "m_dot_MIX", "m_dot_oil", "m_dot_VAP", "m_dot_RES_W", "p_HD", "P_KOMP", "p_ND", "P_PUMP_th", "P_KOMP_th", "Q_dot_ENT", "Q_dot_ENT_W", "Q_dot_oil", "Q_dot_RES_W", "q_geg", "Q_dot_RES", "xi_LIQ", "xi_MIX"] ("Array")) -> (w636:string[])  [unwired: 1 in]
            n121 = property class="Arr (strict)"("Visible"=TRUE) -> ()  [unwired: 2 in, 2 out]
            n122 = Insert Into Array(array=w626, new element=w625) -> (w623:dbl[])  [unwired: 1 in]
            n123 = expression code="x*0.05"(w623) -> (w624:dbl[])
            n124 = Add(x=w623, y=w624) -> (x+y=w632:dbl[])
            n125 = Subtract(x=w623, y=w624) -> (x-y=w631:dbl[])
            n126 = Greater Or Equal?(x=w632, y=w622) -> (x >= y?=w633:bool[])
            n127 = Less Or Equal?(x=w631, y=w622) -> (x <= y?=w634:bool[])
            n128 = And(x=w633, y=w634) -> (x .and. y?=w630:bool[])
            n129 = Build Cluster Array(w623, w622, w636, w630) -> (→"?":T14)
          }
        }
        n130 = Index Array(array=w175, index #1=2 ("index"), index #2=3 ("index"), index #3=4, index #4=5, index #5=11 ("index")) -> (element #1=w242:dbl, element #2=w241:dbl, element #3=w240:dbl, element #4=w246:dbl, element #5=w223:dbl)
        n131 = Build Array(w242, w241, w240) -> (w239:dbl[])
        n132 = Index Array(array=w116, index #1=19, index #2=w365, index #3=w360, index #4=23) -> (element #1=w357:dbl, element #2=w356:dbl, element #3=w355:dbl, element #4=w354:dbl)
        n133 = Index Array(array=w175, index #1=w365, index #2=w360) -> (element #1=w363:dbl, element #2=w362:dbl)
        n134 = Array Max & Min(array=w239) -> (min value=w136:dbl)  [unwired: 3 out]
        n135 = call "Filter5"("Signal"=w362) -> ("Filtered Signal"=w358:dynamicdata)  [unwired: 9 in, 1 out]
        n136 = call "Filter4"("Signal"=w363) -> ("Filtered Signal"=w359:dynamicdata)  [unwired: 9 in, 1 out]
        n137 = Less?(x=w136, y=20.5 ("x")) -> (x < y?=w135:bool)
        n138 = Greater Or Equal?(x=w136, y=18.5 ("x")) -> (x >= y?=w113:bool)
        "Druckzustand" <- w113
        n139 = call "Convert from Dynamic Data11"("Dynamic Data Type"=w359) -> ("Scalar"=w353:dbl)  [unwired: 3 in]
        n140 = call "Convert from Dynamic Data12"("Dynamic Data Type"=w358) -> ("Scalar"=w352:dbl)  [unwired: 3 in]
        n141 = formula code="float32 TIM1; float32 P; float32 H; float32 K;\nH=0; K=0;\nTIM1=((TI36*FI35)+(TI32*FIOel))/(FI35+FIOel);\nif((TI36-TI35) > 2) {\nif((TIM1-TI35) < (0.2)) {\nH=1;}\nelse {\nH=0;}\nif((TI35-TI30) < (0.2)) {\nK=1;}\nelse {\nK=0; }\nP=100/(TIM1-TI30)*(TI35-TI30);\n}"("TI30"=w357, "TI32"=w356, "TI35"=w355, "TI36"=w354, "FIOel"=w353, "FI35"=w352) -> ("H"=w351:sgl, "K"=w348:sgl, "P"=→"%":sgl)  [unwired: 1 out]
        n142 = feedback #1() -> (w127:dbl)  [unwired: 1 in]
        n143 = Select(t=w118, s=w135, f=w127) -> (s? t:f=w128:dbl)
        n144 = feedback-in #1(w128) -> ()
        n145 = case shown="True" "Pumpen-Auto-Abschalt" {
          tunnel: w223 -> [_ w643]
          frame False {
          }
          frame True {
            n146 = Less?(x=w643, y=0.3) -> (x < y?=w642:bool)
            n147 = case shown="True" w642 {
              frame False {
              }
              frame True {
                n148 = local write "Pumpensteuerung"(0.0) -> ()
              }
            }
          }
        }
        n149 = Subtract(x=w118, y=w128) -> (x-y=w134:dbl)
        n150 = Greater Or Equal?(x=w246, y=9.9 ("x")) -> (x >= y?=w250:bool)
        n151 = Greater Or Equal?(x=w134, y=w133) -> (x >= y?=w132:bool)
        n152 = Or(x=w132, y=w250) -> (x .or. y?=w232:bool)
        n153 = Or(x="Drehzahl Bestätigung", y=w232) -> (x .or. y?=w234:bool)
        n154 = case shown="True" w113 {
          frame False {
          }
          frame True {
            n155 = call <vilib>:"Play Sound File.vi"("path"=path "\\\\PCIFT88\\Studenten/Niculovic/LV Spielerei/Ente.wav", "device ID"=u32 0) -> ()  [unwired: 8 in, 2 out]
          }
        }
        n156 = Equal?(x=w351, y=w347) -> (x = y?=→"warm":bool)
        n157 = Equal?(x=w348, y=w347) -> (x = y?=→"kalt":bool)
        n158 = feedback #2() -> (w233:dbl)  [unwired: 1 in]
        "Check" <- w233
        n159 = case shown="True" w232 {
          tunnel: w233 -> [w467 w471]
          tunnel: [w467 w472] -> w140
          frame False {
          }
          frame True {
            n160 = local write "Drehzahl SW"(1000.0) -> ()
            n161 = Multiply(x=w471, y=0.0) -> (x*y=w472:dbl)
            n162 = local write "Regler Hochdruck"(FALSE ("Regler Hochdruck")) -> ()
            n163 = local write "Exp.V"(60.0 ("Exp.V")) -> ()
          }
        }
        n164 = Select(t=0.0, s=w232, f="Drehzahl SW") -> (s? t:f=w236:dbl)
        n165 = feedback-in #2(w236, w234) -> ()
        n166 = local read "Konzentration"() -> (w114:dbl)
        n167 = case shown="True" "Rampe" {
          tunnel: [w423 w424] -> w139
          tunnel: w140 -> [w423 w426]
          frame False {
          }
          frame True {
            n168 = local read "Drehzahl"() -> (w425:dbl)
            n169 = formula code="if (ns > 100) {\nns=100;}\nif (ns < 1) {\nns=1;}\nif ((nSW>nSWR) &&  (nIW>=1000)) {\nnSWR=nSWR+ns;}\nelse {\nnSWR=nSW;}"("nSW"=w426, "ns"="Rampe rpm/s", "nIW"=w425) -> ("nSWR"=w424:dbl)
            "Rampe IW" <- w424
          }
        }
        n170 = case shown="True" "Xi / p_liq berechnung an" {
          tunnel: w116 -> [_ w466]
          tunnel: w175 -> [_ w459]
          tunnel: [0.0 w452] -> w225
          tunnel: [0.0 w449] -> w215
          tunnel: w115 -> [_ w447]
          tunnel: w114 -> [_ w446]
          frame False {
          }
          frame True {
            n171 = Index Array(array=w447, index=8) -> ()  [unwired: 1 out]
            n172 = Index Array(array=w459, index #1=4 ("index"), index #2=8 ("index")) -> (element #1=w454:dbl, element #2=w453:dbl)
            n173 = Index Array(array=w466, index #1=7 ("index"), index #2=6 ("index"), index #3=13 ("index"), index #4=14 ("index"), index #5=5 ("index")) -> (element #1=w458:dbl, element #2=w457:dbl, element #3=w456:dbl, element #4=w455:dbl, element #5=w450:dbl)
            n174 = script code="xi_a = xi_a/100;\ntry\nF = @(xi_r) ((refpropm('H','T',T6a+273.15,'P',p7*100,'ammonia','water',[xi_r 1-xi_r])*0.001-refpropm('H','T',T7+273.15,'P',p7*100,'ammonia','water',[xi_r 1-xi_r])*0.001)/(refpropm('H','T',T14+273.15,'P',p14*100,'ammonia','water',[xi_a 1-xi_a])*0.001-refpropm('H','T',T13+273.15,'P',p14*100,'ammonia','water',[xi_a 1-xi_a])*0.001)*(xi_a-1)+1-xi_r);\nxi_r0=xi_a;\n[xi_r, fval] = fzero(F,xi_r0);\n\np_liq=refpropm('P','T',T6+273.15,'Q',0,'ammonia','water',[xi_r 1-xi_r])/100;\ncatch\nxi_r=1\np_liq=refpropm('P','T',T6+273.15,'Q',0,'ammonia','water',[xi_r 1-xi_r])/100;\nend"("T7"=w458, "T6a"=w457, "T13"=w456, "T14"=w455, "xi_a"=w446, "p7"=w454, "p14"=w453, "T6"=w450) -> ("xi_r"=w452:dbl, "p_liq"=w449:dbl)  [unwired: 1 in, 1 out]
          }
        }
        "xi_r" <- w225
        "p_liq" <- w215
        n175 = Index Array(array=w175, index=13) -> (element=w177:dbl)
        n176 = Index Array(array=w116, index=22) -> (element=w150:dbl)
        n177 = call "Filter9"("Signal"=w215) -> ("Filtered Signal"=w213:dynamicdata)  [unwired: 9 in, 1 out]
        "p_liq_mittel" <- w213
        n178 = call "Pumpensteuerung_PID.vi"("reinitialize? (F)"="reinitialize Pumpe", "PID Regelung Pumpe"="PID Regelung Pumpe", "FI13 SW in l/min"="FI13 SW in l/min", "Prozessvariable"=w177, "Pumpensteuerung"="Pumpensteuerung") -> ("upper limit"=w220:dbl)  [unwired: 4 in, 2 out]
        n179 = call "Senkenregler_PID.vi"("Regelventil 36"="Regelventil 36", "Solltemp."="TI35 SW", "Regelventil 35"="Regelventil 35", "Regler Senke"="Regler Senke", "reinitialize?"="reinitialize Senke", "TI_35"=w150) -> ("upper limit 2"=w229:dbl, "upper limit"=w227:dbl)  [unwired: 6 in, 2 out]
        n180 = Greater?(x=w213, y=15.0) -> (0:w212:dynamicdata)
        n181 = case shown="True" w212 {
          tunnel: [w438 15.0 ("y")] -> w211
          tunnel: w212 -> [w438 _]
          frame False {
          }
          frame True {
          }
        }
        n182 = call "Filter7"("Signal"=w220) -> ("Filtered Signal"=w219:dynamicdata)  [unwired: 9 in, 1 out]
        "Mittelwert" <- w219
        n183 = Add(x="zusätzlicher Druck", y=w211) -> (x+y=w210:dynamicdata)
        n184 = case shown="True" "Mittelwert Pumpe" {
          tunnel: w220 -> [w442 _]
          tunnel: [w442 w443] -> w221
          tunnel: w219 -> [_ w443]
          frame False {
          }
          frame True {
          }
        }
        n185 = Greater Than 0?(x="RV 33") -> (x > 0?=w256:bool)
        n186 = Less Than 0?(x="RV 33") -> (x < 0?=w255:bool)
        n187 = Select(t=w391, s=w255, f=w392) -> (s? t:f=w389:i32)
        n188 = Select(t=w391, s=w256, f=w392) -> (s? t:f=w390:i32)
        n189 = call "Hochdruckregler_PID.vi"("Regler Hochdruck"="Regler Hochdruck", "Steuereingang"=w210, "Solldruck"="PI05 SW", "PI05"=w175, "Exp.V"="Exp.V", "reinitialize? (F) in"="reinitialize HD") -> ("upper limit out"=w152:dbl)  [unwired: 7 in, 2 out]
        n190 = call "Filter8"("Signal"=w152) -> ("Filtered Signal"=w216:dynamicdata)  [unwired: 9 in, 1 out]
        "Mittelwert 2" <- w216
        n191 = case shown="True" "Mittelwert HD" {
          tunnel: w152 -> [w440 _]
          tunnel: [w440 w441] -> w217
          tunnel: w216 -> [_ w441]
          frame False {
          }
          frame True {
          }
        }
        n192 = call "Stellungen_Namen2.vi"("Kühlventil"=w229, "Pumpensteuerung"=w221, "Regelventil 39"="Regelventil 39", "Exp.V"=w217, "Regelventil 14"=w227, "Meter"=w139, "zu"="RV 30 zu", "auf"="RV 30 auf", "Regelventil 34"="Regelventil 34") -> ("Dynamic Data"=w287:dynamicdata)  [unwired: 2 in]
        n193 = Build Array("PI05 SW", "TI35 SW", "FI13 SW in l/min") -> (w146:dbl[])
        n194 = Merge Signals(w287, w390, w389) -> (w153:dynamicdata)
        n195 = Insert Into Array(array=w115, new element=w146) -> (w117:dbl[])  [unwired: 1 in]
        n196 = call-poly <vilib>:"DAQmx Write.vi"("task/channels in"=w155, "auto start"=w156, "data"=w153, "error in"=w154) -> ()  [unwired: 9 in, 3 out]
        n197 = Index Array(array=w116, index=18) -> (element=w279:dbl)
        n198 = Index Array(array=w175, index #1=1, index #2=0, index #3=7, index #4=6) -> (element #1=w276:dbl, element #2=w275:dbl, element #3=w274:dbl, element #4=w273:dbl)
        n199 = Index Array(array=w117, index=0) -> (element=w208:dbl)
        n200 = Not Equal To 0?(x=w208) -> (x != 0?=w126:bool)
        n201 = Divide(x=w276, y=w275) -> (x/y=w397:dbl)
        "Druckverhältnis" <- w397
        n202 = Subtract(x=w274, y=w273) -> (x-y=w407:dbl)
        n203 = Greater?(x=w407, y=1.0) -> (0:w281:bool)
        "Fl.Pumpe an" <- w281
        n204 = feedback #3() -> (w124:dbl)  [unwired: 1 in]
        n205 = Select(t=w124, s=w126, f=w118) -> (s? t:f=w125:dbl)
        n206 = feedback-in #3(w125) -> ()
        n207 = Less?(x=w279, y=60) -> (x < y?=w343:bool)
        "Temperatur Öl" <- w343
        n208 = Greater?(x=w397, y=1.5) -> (0:w395:bool)
        n209 = feedback #4(w118) -> (w119:dbl)
        n210 = Select(t=w118, s="Reset", f=w119) -> (s? t:f=w120:dbl)
        n211 = feedback-in #4(w120) -> ()
        n212 = Subtract(x=w118, y=w125) -> (x-y=w123:dbl)
        n213 = Subtract(x=w118, y=w120) -> (x-y=w122:dbl)
        n214 = expression code="x-3600"(w123) -> (w400:dbl)
        n215 = Build Array(w343, w395) -> (→"Warnungen":bool[])
        n216 = expression code="x-3600"(w122) -> (w402:dbl)
        n217 = Greater?(x=w123, y=720.0) -> (0:w282:bool)
        "Magnetventil" <- w282
        n218 = Build Array(w126, w282, w281) -> (→"Status Komponenten":bool[])
        n219 = call "Verdichternamen.vi"("Array"=w117) -> ("Dynamic Data"=w398:dynamicdata)  [unwired: 10 in]
        n220 = Seconds To Date/Time(time stamp (now)=w400) -> (date time rec=w344:T15)  [unwired: 1 in]
        n221 = Seconds To Date/Time(time stamp (now)=w402) -> (date time rec=w411:T15)  [unwired: 1 in]
        n222 = Unbundle By Name(w411) -> ("second"=w410:i32, "minute"=w409:i32, "hour"=w403:i32)
        n223 = Unbundle By Name(w344) -> ("second"=w413:i32, "minute"=w412:i32, "hour"=w401:i32)
        n224 = Bundle("second"=w413, "minute"=w412, "hour"=w401) -> (→"Verdichteraktivität":cluster{"second":i32, "minute":i32, "hour":i32})  [unwired: 1 in]
        n225 = Bundle("second"=w410, "minute"=w409, "hour"=w403) -> (→"Betriebszeit":cluster{"second":i32, "minute":i32, "hour":i32})  [unwired: 1 in]
        n226 = local read "Array 2"() -> (w112:waveform(dbl)[])
        n227 = Merge Signals(w170, w169, w287, w398, w112) -> (w306:dynamicdata)
        n228 = flat-sequence {
          tunnel: [w501] -> w420
          tunnel: [w500] -> w419
          tunnel: w324 -> [w499]
          tunnel: w323 -> [w498]
          tunnel: [w496] -> w320
          tunnel: "Identität!" -> [w495]
          tunnel: "Dateiname!" -> [w494]
          tunnel: "Speichern" -> [w493]
          tunnel: "tag" -> [w492]
          tunnel: w420 -> [w599]
          tunnel: w419 -> [w598]
          tunnel: [w594] -> w327
          tunnel: [w596] -> w326
          tunnel: w325 -> [w595]
          frame #0 {
            n229 = Index Array(array=w498) -> (element=w497:timestamp)  [unwired: 1 in]
            n230 = event shown="[1] \"Speichern\": Value Change" {
              selector: _ -> [_ _ _]
              dyn-events: _ -> [_ _ _]
              timeout: 5 -> [_ _ _]
              tunnel: [_ w511 _] -> w501
              tunnel: w499 -> [_ w506 _]
              tunnel: ["" w510 ""] -> w500
              tunnel: w497 -> [_ w509 w580]
              tunnel: [_ _ w578] -> w496
              tunnel: w495 -> [_ w508 _]
              tunnel: w494 -> [_ w507 _]
              tunnel: w493 -> [_ w505 _]
              tunnel: w492 -> [_ w504 _]
              event Timeout {
                n231 = event-data() -> ()  [unwired: 1 in, 1 out]
              }
              event "Speichern": Value Change {
                n232 = event-data() -> ()  [unwired: 1 in, 1 out]
                n233 = case shown="True" w505 {
                  tunnel: [w543 _] -> w511
                  tunnel: [w538 _] -> w510
                  tunnel: w509 -> [w530 _]
                  tunnel: w508 -> [w514 _]
                  tunnel: w507 -> [w526 _]
                  tunnel: w506 -> [w525 _]
                  tunnel: w504 -> [w513 _]
                  frame False {
                    w517 = "\r"
                    n234 = property on="Dateiname!" class="Str"("DisabledEnum"=T4."Disabled and Grayed Out" ("Disabled")) -> ()  [unwired: 2 in, 2 out]
                    n235 = for {
                      N: 1 -> [_]
                      tunnel: ["Zeit"] -> w523 mode=indexing
                      tunnel: ["Kommentar"] -> w519 mode=indexing
                    }
                    n236 = Format Date/Time String(time format string (%c)="%d-%m-%Y_%H.%M ", seconds (now)=w530) -> (date/time string=w531:string)  [unwired: 1 in]
                    n237 = Concatenate Strings(w514, "\\", w531, w526, ".lvm" ("string")) -> (w533:string)
                    n238 = Insert Into Array(array=w525, index (row)=0, new element=w523) -> (w521:string[][])  [unwired: 1 in]
                    n239 = Build Path(base path=path "\\\\pcift88\\Studenten/HT-Waermepumpe/Messdaten" ("file path (dialog if empty)"), name or relative path=w533) -> (appended path=w528:path)
                    n240 = Concatenate Strings(w514, "\t", "tag: " ("string"), w513) -> (w512:string)
                    n241 = Insert Into Array(array=w521, new element=w519) -> (w520:string[][])  [unwired: 2 in]
                    n242 = Open/Create/Replace File(file path (use dialog)=w528, operation (0:open)=T11."replace or create with confirmation") -> (refnum out=→"refnum out":refnum<file>, error out=w543:errorcluster)  [unwired: 4 in, 1 out]
                    n243 = Transpose 2D Array(2D array=w520) -> (transposed array=w541:string[][])
                    n244 = Format Date/Time String(seconds (now)=w530) -> (date/time string=w540:string)  [unwired: 2 in]
                    n245 = Strip Path(path=w528) -> (name=w527:string)  [unwired: 1 out]
                    n246 = Array To Spreadsheet String(array=w541, 3:"%s" ("format string")) -> (spreadsheet string=w539:string)  [unwired: 1 in]
                    n247 = Concatenate Strings(w512, w517, w517, w527, w517, w517, w540, w517, w517, w539, w517, w517) -> (w538:string)
                  }
                  frame True {
                    n248 = local read "refnum out"() -> (w547:refnum<file>)
                    n249 = property on="Dateiname!" class="Str"("DisabledEnum"=T4."Enabled" ("Disabled")) -> ()  [unwired: 2 in, 2 out]
                    n250 = Close File(refnum=w547) -> ()  [unwired: 1 in, 2 out]
                  }
                }
              }
              event "Comment": Value Change {
                # "Umlaute + ß ersetzen, quick&dirty 4.1.2016"
                n251 = event-data() -> ()  [unwired: 1 in, 1 out]
                n252 = flat-sequence {
                  tunnel: ["Kommentar"] -> w548
                  tunnel: w580 -> [w584]
                  frame #0 {
                    w586 = "\r"
                    n253 = local read "Historie"() -> (w588:string)
                    n254 = Get Date/Time String(seconds (now)=w584, want seconds? (F)=TRUE) -> (time string=w587:string)  [unwired: 1 in, 1 out]
                    n255 = Concatenate Strings(w588, w587, " -> ", "Kommentar", w586, w586) -> (→"Historie":string)
                  }
                  frame #1 {
                    n256 = local write "Kommentar"("") -> ()
                  }
                }
                n257 = Search and Replace String(replace all?=TRUE, input string=w548, search string="ä", replace string="ae") -> (result string=w570:string)  [unwired: 4 in, 3 out]
                n258 = Search and Replace String(replace all?=TRUE, input string=w570, search string="ü", replace string="ue") -> (result string=w569:string)  [unwired: 4 in, 3 out]
                n259 = Search and Replace String(replace all?=TRUE, input string=w569, search string="ö", replace string="oe") -> (result string=w568:string)  [unwired: 4 in, 3 out]
                n260 = Search and Replace String(replace all?=TRUE, input string=w568, search string="ß", replace string="ss") -> (result string=w549:string)  [unwired: 4 in, 3 out]
                n261 = Search and Replace String(replace all?=TRUE, input string=w549, search string="Ä", replace string="Ae") -> (result string=w558:string)  [unwired: 4 in, 3 out]
                n262 = Search and Replace String(replace all?=TRUE, input string=w558, search string="Ü", replace string="Ue") -> (result string=w557:string)  [unwired: 4 in, 3 out]
                n263 = Search and Replace String(replace all?=TRUE, input string=w557, search string="Ö", replace string="Oe") -> (result string=w550:string)  [unwired: 4 in, 3 out]
                n264 = for {
                  N: 1 -> [_]
                  tunnel: [w581] -> w578 mode=indexing
                  tunnel: w550 -> [w581]
                }
              }
            }
          }
          frame #1 {
            n265 = local read "refnum out"() -> (w591:refnum<file>)
            n266 = Concatenate Strings(w598, w595) -> (w597:string)
            n267 = Not A Number/Path/Refnum?(number/path/refnum=w591) -> (NaN/Path/Refnum?=w592:bool)
            n268 = Set File Position(refnum=w591, from (0:start)=enum16{"start", "end", "current"}."end", error in=w599) -> (refnum out=w600:refnum<file>, error out=w601:errorcluster)  [unwired: 1 in]
            n269 = Not(x=w592) -> (.not. x?=→"Speichert!":bool)
            n270 = Write to Text File(file (use dialog)=w600, text=w597, error in=w601) -> (refnum out=w594:refnum<file>, error out=w596:errorcluster)  [unwired: 1 in, 1 out]
          }
        }
        n271 = Empty String/Path?(string/path="Identität!") -> (empty?=w318:bool)
        n272 = Empty String/Path?(string/path="Dateiname!") -> (empty?=w317:bool)
        n273 = Or(x=w318, y=w317) -> (x .or. y?=w314:bool)
        n274 = call "Protokollordnung"("Signals"=w306) -> ("Signal Out"=w332:dynamicdata)  [unwired: 9 in, 1 out]
        n275 = Boolean To (0,1)(Boolean=w314) -> (0, 1=w315:i16)
        n276 = expression code="x*2"(w315) -> (w316:i16)
        n277 = property on="Speichern" class="Bool (strict)"("DisabledEnum"=w316) -> ()  [unwired: 2 in, 2 out]
        n278 = call "Convert from Dynamic Data"("Dynamic Data Type"=w332) -> ("Array of Waveform"=w333:waveform(dbl)[])  [unwired: 3 in]
        n279 = Array Size(array=w333) -> (size(s)=w310:i32)
        n280 = Concatenate Strings("%" ("string"), "." ("string"), ";%g" ("string")) -> (w335:string)
        n281 = Initialize Array(w335, w310) -> (w334:string[])
        n282 = for {
          tunnel: w333 -> [w605] mode=indexing
          tunnel: [w612] -> w330 mode=indexing
          tunnel: w334 -> [w610] mode=indexing
          tunnel: [w604] -> w324 mode=indexing
          tunnel: [w606] -> w323 mode=indexing
          tunnel: [w607] -> w329 mode=indexing
          n283 = Unbundle By Name(w605) -> ("Y"=w611:dbl[], "t0"=w603:timestamp)
          n284 = Get Waveform Attribute(5:w603, 6:"NI_ExpTimeStamp", 7:w605) -> (1:w606:timestamp)  [unwired: 1 in, 3 out]
          n285 = for {
            tunnel: w611 -> [w619] mode=indexing
            tunnel: [w618] -> w612 mode=indexing
            tunnel: w610 -> [w617]
            tunnel: w605 -> [w616]
            tunnel: [w615] -> w604 mode=indexing
            n286 = Format Into String(format string=w617, w619) -> (resulting string=w618:string)  [unwired: 2 in, 1 out]
            n287 = Get Waveform Attribute(5:"", 6:"NI_ChannelName", 7:w616) -> (1:w615:string)  [unwired: 1 in, 3 out]
          }
          n288 = Format Date/Time String(time format string (%c)="%H.%M.%S", seconds (now)=w606) -> (date/time string=w607:string)  [unwired: 1 in]
        }
        n289 = Insert Into Array(array=w330, index (row)=0, new element=w329) -> (w321:string[][])  [unwired: 1 in]
        n290 = Increment(x=w310) -> (x+1=w311:i32)
        n291 = Insert Into Array(array=w321, index (row)=w311, new element=w320) -> (w322:string[][])  [unwired: 1 in]
        n292 = Transpose 2D Array(2D array=w322) -> (transposed array=w319:string[][])
        n293 = Array To Spreadsheet String(array=w319, 3:"%s" ("format string")) -> (spreadsheet string=w325:string)  [unwired: 1 in]
      }
      frame #2 {
        n294 = Tick Count (ms)() -> (millisecond timer value=w737:u32)
        n295 = Subtract(x=w737, y=w736) -> (x-y=w735:u32)
        n296 = Divide(x=w735, y=1000.0) -> (x/y=→"Schleifendauer":dbl)
      }
    }
  }
  n297 = while {
    tunnel: w4 -> [w752]
    tunnel: w3 -> [w751]
    tunnel: w7 -> [w750]
    stop <- w743 stop-if-true
    n298 = flat-sequence {
      tunnel: [w778] -> w770
      tunnel: w751 -> [w775]
      tunnel: [w780] -> w769
      tunnel: w750 -> [w778]
      tunnel: w752 -> [w779]
      tunnel: [w774] -> w745
      tunnel: w770 -> [w784]
      tunnel: [w784] -> w768
      tunnel: [w783] -> w767
      tunnel: w769 -> [w783]
      tunnel: w745 -> [w782]
      tunnel: [w782] -> w744
      tunnel: w768 -> [w788]
      tunnel: [w788] -> w766
      tunnel: w767 -> [w790]
      tunnel: [w789] -> w765
      tunnel: [w787] -> w746
      tunnel: w744 -> [w786]
      tunnel: w766 -> [w794]
      tunnel: [w794] -> w764
      tunnel: w765 -> [w793]
      tunnel: [w793] -> w763
      tunnel: [w792] -> w747
      tunnel: w746 -> [w792]
      tunnel: w764 -> [w797]
      tunnel: [w797] -> w762
      tunnel: [w801] -> w761
      tunnel: [w800] -> w760
      tunnel: [w799] -> w759
      tunnel: w763 -> [w796]
      tunnel: w747 -> [w795]
      tunnel: w762 -> [w807]
      tunnel: [w806] -> w740
      tunnel: w761 -> [w805]
      tunnel: w760 -> [w804]
      tunnel: w759 -> [w808]
      tunnel: [w805] -> w754
      tunnel: [w804] -> w753
      frame #0 {
        n299 = Format Into String(format string="%.0f", w778) -> (resulting string=w773:string)  [unwired: 2 in, 1 out]
        n300 = Concatenate Strings("TRAC:CLE:AUTO ON\nTRAC:POIN ", w773, "\nTRAC:FEED SENS\nTRAC:FEED:CONT NEXT\nINIT\n" ("Daten")) -> (w771:string)
        n301 = VISA Write(VISA resource name=w779, write buffer=w771, error in (no error)=w775) -> (VISA resource name out=w780:refnum<visa-resource-name>, error out=w774:errorcluster)  [unwired: 1 out]
      }
      frame #1 {
        (unwired) u32 1600 ("ms Wartezeit")
        n302 = Wait (ms)(milliseconds to wait="Wartezeit 1") -> ()  [unwired: 1 out]
      }
      frame #2 {
        n303 = VISA Write(VISA resource name=w790, write buffer="FORM:ELEM READ\nTRAC:DATA?\n", error in (no error)=w786) -> (VISA resource name out=w789:refnum<visa-resource-name>, error out=w787:errorcluster)  [unwired: 1 out]
      }
      frame #3 {
        (unwired) u32 200 ("ms Wartezeit")
        n304 = Wait (ms)(milliseconds to wait="Wartezeit 2") -> ()  [unwired: 1 out]
      }
      frame #4 {
        n305 = property class="Instr"(reference=w796, error in=w795) -> (reference out=w802:refnum<visa-resource-name>, error out=w803:errorcluster, "Bytes at Port"=w798:u32)
        n306 = VISA Read(VISA resource name=w802, byte count=w798, error in (no error)=w803) -> (VISA resource name out=w801:refnum<visa-resource-name>, read buffer=w799:string, error out=w800:errorcluster)  [unwired: 1 out]
      }
      frame #5 {
        n307 = Initialize Array(0.0 ("Elementdaten"), w807) -> (w813:dbl[])
        n308 = Concatenate Strings(w808, "," ("Sub-Sring")) -> (w810:string)
        n309 = for {
          N: w807 -> [_]
          shift-right: [w823] -> w806
          shift-left: w813 -> [w814]
          shift-right: [w816] -> _
          shift-left: w810 -> [w822]
          shift-right: [w817] -> _
          shift-left: 0 -> [w818]
          n310 = Increment(x=w818) -> (x+1=w817:i32)
          n311 = Match Pattern(string=w822, regular expression="," ("gültiger Ausdruck")) -> (before substring=w819:string, after substring=w816:string)  [unwired: 1 in, 2 out]
          n312 = Fract/Exp String To Number(use system decimal point (T)=FALSE ("verwende System-Dezimalpunkt (T)"), string=w819) -> (number=w820:dbl)  [unwired: 2 in, 1 out]
          n313 = Replace Array Subset(array=w814, new element=w820, index=w818) -> (w823:dbl[])
        }
      }
    }
    n314 = VISA Close(VISA resource name=w754, error in (no error)=w753) -> ()  [unwired: 1 out]
    n315 = call "Messplattenanzeige.vi"("Array"=w740) -> ()  [unwired: 11 in]
    n316 = formula code="a[0]=1001;\na[1]=1001;\na[2]=1001;\na[3]=1001;\na[4]=1001;\na[5]=1001;\na[6]=1001;\na[7]=1001;\na[8]=1001;\na[9]=1001;\na[10]=1001;\na[11]=1001;\na[12]=1001;\na[13]=1001;\na[14]=1001;\na[15]=1001;\na[16]=1001;\na[17]=1001;\na[18]=1001;\na[19]=1001;\na[20]=1001;\na[21]=1001;\na[22]=1001;\na[23]=1001;\na[24]=1001;\na[25]=1001;\na[26]=1001;\na[27]=1001;\na[28]=1001;\na[29]=1001;\na[30]=1001;\na[31]=1001;\na[32]=1001;\na[33]=1001;\na[34]=1001;\na[35]=1001;\na[36]=1001;\na[37]=1001;\na[38]=1001;\na[39]=1001;\na[40]=1001;\na[41]=1001;\na[42]=1001;\na[43]=1001;\na[44]=1001;\na[45]=1001;\na[46]=1001;\na[47]=1001;\na[48]=1001;\na[49]=1001;\na[50]=1001;"("a"=w740) -> ()  [unwired: 1 out]
    n317 = Get Date/Time In Seconds() -> (seconds since 1Jan1904=w749:timestamp)
    n318 = Spreadsheet String To Array(delimiter (Tab)=",", format string="%.3f", spreadsheet string="TC 101,TC 102,TC 103,TC 104,TC 105,TC 106,TC 107,TC 108,TC 109,TC 110,TC 111,TC 112,TC 113,TC 114,TC 115,TC 116,TC 117,TC 118,TC 119,TC 120,TC 121,TC 122,TC 123,TC 124,TC 125,TC 126,TC 127,TC 128,TC 129,TC 130,TC 131,TC 132,TC 133,TC 134,TC 135,TC 136,TC 137,TC 138,TC 139,TC 140,TC 201,TC 202,TC 203,TC 204,TC 205,TC 206,TC 207,TC 208,TC 209,TC 210,TC 211,TC 212,TC 213,TC 214,TC 215,TC 216,TC 217,TC 218,TC 219,TC 220,TC 221,TC 222,TC 223,TC 224,TC 225,TC 226,TC 227,TC 228,TC 229,TC 230,TC 231,TC 232,TC 233,TC 234,TC 235,TC 236,TC 237,TC 238,TC 239,TC 240,TC 301,TC 302,TC 303,TC 304,TC 305,TC 306,TC 307,TC 308,TC 309,TC 310,TC 311,TC 312,TC 313,TC 314,TC 315,TC 316,TC 317,TC 318,TC 319,TC 320,TC 401,TC 402,TC 403,TC 404,TC 405,TC 406,TC 407,TC 408,TC 409,TC 410,TC 411,TC 412,TC 413,TC 414,TC 415,TC 416,TC 417,TC 418,TC 419,TC 420", array type (2D Dbl)=string[] []) -> (array=w757:string[])
    n319 = for {
      tunnel: w757 -> [w829] mode=indexing
      tunnel: [w826] -> w741 mode=indexing
      tunnel: w749 -> [w825]
      tunnel: w740 -> [w824] mode=indexing
      n320 = Build Array(w824) -> (w828:dbl[])
      n321 = Bundle By Name("Y"=w828, "t0"=w825) -> (w827:waveform(dbl))  [unwired: 1 in]
      n322 = Set Waveform Attribute(5:w829, 6:"NI_ChannelName", 7:w827) -> (3:w826:waveform(dbl))  [unwired: 1 in, 2 out]
    }
    "Array 2" <- w741
    n323 = local read "Programm stoppen!"() -> (w743:bool)
    n324 = call "Write To Measurement File"("Signals"=w741, "Enable"="Messplatten speichern") -> ()  [unwired: 15 in, 3 out]
  }
  n325 = call <vilib>:"DAQmx Clear Task.vi"("task in"=w16, "error in"=w14) -> ()  [unwired: 13 in, 1 out]
  n326 = call <vilib>:"DAQmx Clear Task.vi"("task in"=w15, "error in"=w13) -> ()  [unwired: 13 in, 1 out]
  n327 = Close File(refnum=w41, error in=w40) -> (error out=w44:errorcluster)  [unwired: 1 out]
  n328 = call <vilib>:"General Error Handler.vi"("error in (no error)"=w44, "[exception action] (none:0)"=1 ("[exception code]"), "[exception code]"=1) -> ()  [unwired: 8 in, 5 out]
